vi "GFITS_LibSetNzim.vi"(8 "error in (no error)":errorcluster, 10 "n z images":u32=1) -> (0 "error out":errorcluster, 2 "return value":i32)   [LabVIEW 2016]
uses:
  c/lib/libgfits.so
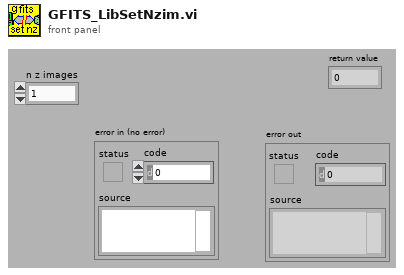
[diagram p1: front panel]
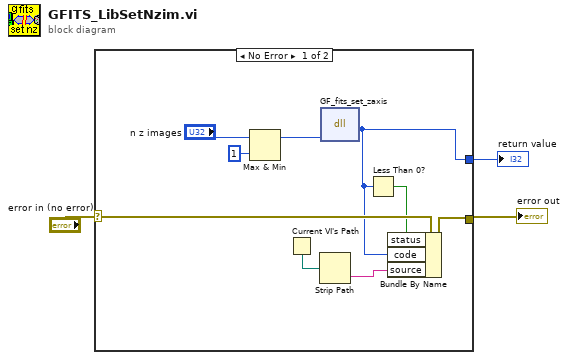
[diagram p0: block diagram]
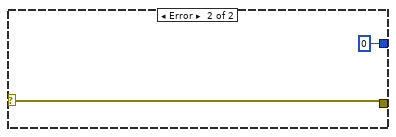
[diagram p2: hidden frame]
diagram:
  n1 = case shown="No Error" "error in (no error)" {
    selector: "error in (no error)" -> [w12 w14]
    tunnel: [w10 0] -> w3
    tunnel: [w7 w14] -> w1
    frame No Error {
      n2 = Max & Min(x="n z images", y=u32 1) -> (max(x,y)=w4:u32)  [unwired: 1 out]
      n3 = Current VI's Path() -> (path=w9:path)
      n4 = Strip Path(path=w9) -> (name=w8:string)  [unwired: 1 out]
      n5 = dll-call lib="home/simager/panview/PAN/Modules/GFITS/private/c/lib/libgfits.so" fn="GF_fits_set_zaxis"("nz"=w4) -> ("return type"=w10:i32)  [unwired: 4 in, 2 out]
      n6 = Less Than 0?(x=w10) -> (x < 0?=w11:bool)
      n7 = Bundle By Name(cluster=w12, "status"=w11, "code"=w10, "source"=w8) -> (w7:errorcluster)
    }
    frame Error {
    }
  }
  "return value" <- w3
  "error out" <- w1
